vi "WindGoodnessAtHeading.vi"(10 "Wind Direction":i32, 11 "Heading":i32) -> (3 "Wind goodness\nat this heading":sgl)   [LabVIEW 2011]
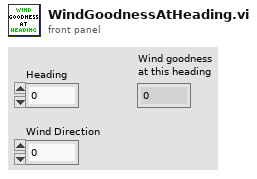
[diagram p1: front panel]
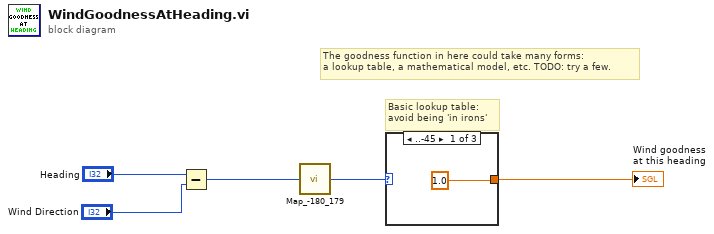
[diagram p0: block diagram]
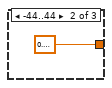
[diagram p2: hidden frame]
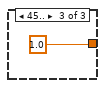
[diagram p3: hidden frame]
diagram:
  # "Basic lookup table:\navoid being 'in irons'"
  # "The goodness function in here could take many forms:\na lookup table, a mathematical model, etc. TODO: try a few."
  n1 = Subtract(x="Heading", y="Wind Direction") -> (x-y=w2:i32)
  n2 = call "Map_-180_179.vi"("Angle In"=w2) -> ("-180 <= Angle out <180"=w1:i32)
  n3 = case shown="..-45" w1 {
    tunnel: [sgl 1.0 sgl 0.1 sgl 1.0] -> w3
    frame ..-45 {
    }
    frame -44..44 {
    }
    frame 45.. {
    }
  }
  "Wind goodness\nat this heading" <- w3
